vi "Pid_v20.vi"() -> ()   [LabVIEW 2020]
doc: "This example demonstrates how to simulate a general PID controller."
uses:
  <vilib>/addons/control/pid/pid.llb/PID (DBL).vi
  <vilib>/addons/control/pid/NI_PID_pid.lvlib
panel:
  in  "r - Set point":dbl(slide)=4.965034965034965 scale=0.0..10.0
  out "y - Iesirea":dbl(slide)=0.4195804195804196 scale=0.0..10.0
  out "u":dbl(slide)=0.27972027972027974 scale=0.0..10.0
  out "U - comanda":dbl(graph)=4.96503496506626
  in  "PID gains":T1={"proportional gain (Kc)"=20.0, "integral time (Ti, min)"=0.008, "derivative time (Td, min)"=0.001} {"derivative time (Td, min)" format="%.3f"; "integral time (Ti, min)" format="%.3f"; "proportional gain (Kc)" format="%.3f"}
  in  "Stop":bool
  out "u,y,r":T2(graph)={"Plant Output"=4.96503496506626, "output"=4.965034965036714, "r - Set point"=4.965034965034965}
  # "Overview: This example demonstrates how to simulate a simple PID loop controller.\nInstructions:\n1. Run the VI and observe the Process variable (PV) following the Setpoint (SP) value while the output of the controller, also called Manipulated variable (MV), changes to keep both values near each other.\n2. After it settles down (value of PV and SP are near each other), change SP. You can just move the 'blue' arrow on the indicator. The MV will change to drive PV to SP again.\n3. Click Stop to stop the VI."
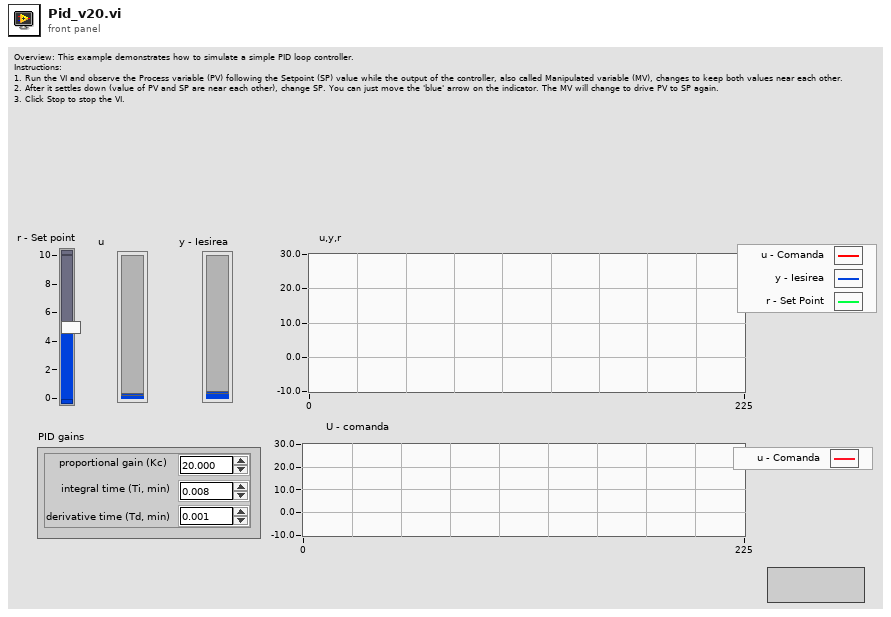
[diagram p1: front panel]
types:
  T1 = cluster{"proportional gain (Kc)":dbl, "integral time (Ti, min)":dbl, "derivative time (Td, min)":dbl}
  T2 = cluster{"Plant Output":dbl, "output":dbl, "r - Set point":dbl}
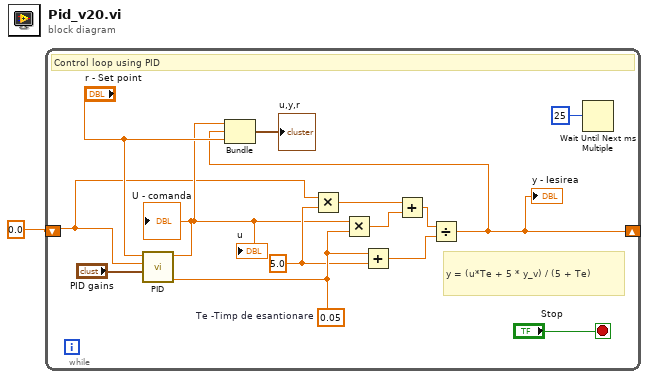
[diagram p0: block diagram]
diagram:
  n1 = while {
    shift-left: 0.0 ("Plant Output") -> [w4]
    shift-right: [w2] -> _
    stop <- "Stop" stop-if-true
    w7 = 5.0 ("y")
    w8 = 0.05  # Te -Timp de esantionare
    # "y = (u*Te + 5 * y_v) / (5 + Te)"
    # "Control loop using PID"
    n2 = call-poly <vilib>:"PID.vi"("dt (s)"=w8, "PID gains"="PID gains", "process variable"=w4, "setpoint"="r - Set point") -> ("output"=w5:dbl)  [unwired: 6 in, 1 out]
    "U - comanda" <- w5
    "u" <- w5
    n3 = Multiply(x=w4, y=w7) -> (x*y=w10:dbl)
    n4 = Multiply(x=w5, y=w8) -> (x*y=w11:dbl)
    n5 = Add(x=w8, y=w7) -> (x+y=w9:dbl)
    n6 = Add(x=w10, y=w11) -> (x+y=w12:dbl)
    n7 = Divide(x=w12, y=w9) -> (x/y=w2:dbl)
    "y - Iesirea" <- w2
    n8 = Bundle("output"=w5, w2, "r - Set point"="r - Set point") -> (→"u,y,r":cluster{"output":dbl, dbl, "r - Set point":dbl})  [unwired: 1 in]
    n9 = Wait Until Next ms Multiple(millisecond multiple=u32 25 ("unsigned 32bit integer")) -> ()  [unwired: 1 out]
  }
